vi "identifying_number.vi"() -> (2 "identifying number":string)   [LabVIEW 2019]
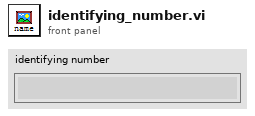
[diagram p1: front panel]
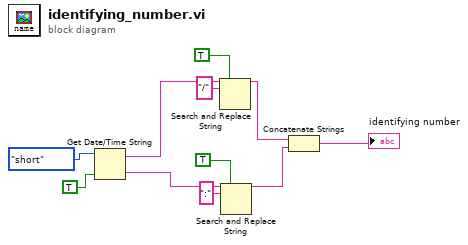
[diagram p0: block diagram]
diagram:
  n1 = Get Date/Time String(date format (0)=enum16{"short", "long", "abbreviated"}."short" ("日期格式(0)"), want seconds? (F)=TRUE ("需要秒？(F)")) -> (date string=w9:string, time string=w6:string)  [unwired: 1 in]
  n2 = Search and Replace String(replace all?=TRUE ("替换全部？(F)"), input string=w9, search string="/" ("搜索字符串")) -> (result string=w3:string)  [unwired: 5 in, 3 out]
  n3 = Search and Replace String(replace all?=TRUE ("替换全部？(F)"), input string=w6, search string=":" ("搜索字符串")) -> (result string=w2:string)  [unwired: 5 in, 3 out]
  n4 = Concatenate Strings(w3, w2) -> (→"identifying number":string)
